vi "Receive String.vi"(8 "error in (no error)":errorcluster, 10 "Broadcast String Msg":refnum<class "Broadcast String Msg.lvclass">, 11 "TopLevelApplication In":refnum<class "TopLevelApplication.lvclass">) -> (0 "error out":errorcluster, 3 "TopLevelApplication Out":refnum<class "TopLevelApplication.lvclass">)   [LabVIEW 2015, in "TopLevelApplication.lvlib" / "TopLevelApplication.lvclass"]
uses:
  TopLevelApplication.lvclass
  IViewable/IViewable Messages/Broadcast String Msg/Broadcast String Msg.lvclass
  IViewable/IViewable Messages/Broadcast String Msg/Broadcast String Msg.lvclass/Broadcast String Msg.ctl
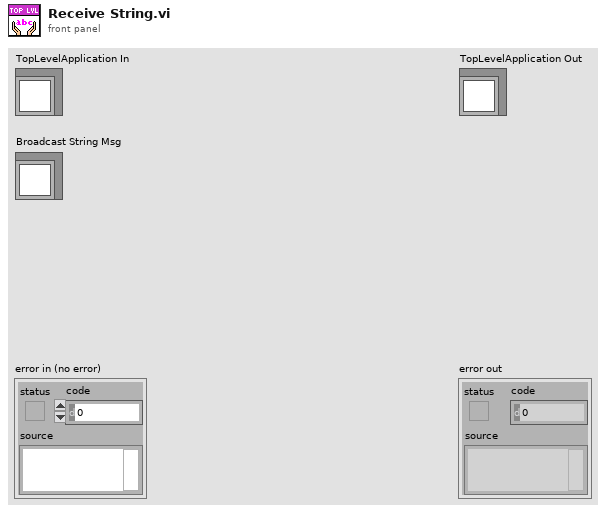
[diagram p1: front panel]
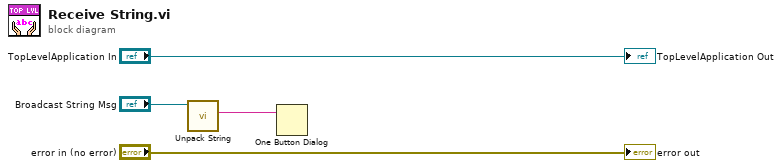
[diagram p0: block diagram]
diagram:
  n1 = call "Unpack String.vi"("Broadcast String Msg In"="Broadcast String Msg") -> ("Value"=w1:string)  [unwired: 9 in, 1 out]
  n2 = One Button Dialog(message=w1) -> ()  [unwired: 1 in, 1 out]
  "error out" <- "error in (no error)"
  "TopLevelApplication Out" <- "TopLevelApplication In"
